vi "Linux parse ip route get.vi"(8 "error in (no error)":errorcluster, 11 "ip route get output":string="192.168.1.5 dev br0 src 192.168.1.100 uid 1000\n     cache") -> (0 "error out":errorcluster, 2 "gw":refnum<class "Generic Network Address.lvclass">, 3 "route ok?":bool)   [LabVIEW 2020, in "NI_WFCN.lvlib" / "IPv4 Network Address.lvclass"]
doc: "Linux: Parse the output of `ip route get $ip` to determine if an address is routable."
uses:
  <vilib>/net/WFCN/Addressing/IPv4 Network Address/IPv4 Network Address.lvclass
  <vilib>/net/WFCN/Addressing/Generic Network Address/Generic Network Address.lvclass
  <vilib>/net/WFCN/Addressing/IPv4 Network Address/IPv4 Network Address.lvclass/IPv4 Network Address.ctl
  <vilib>/net/WFCN/Addressing/Generic Network Address/Generic Network Address.lvclass/Generic Network Address.ctl
  <vilib>/net/WFCN/Addressing/Hostname Network Address/Hostname Network Address.lvclass/Hostname Network Address.ctl
  <vilib>/net/WFCN/Addressing/Hostname Network Address/Create from string.vi
  <vilib>/net/WFCN/Utility/Is IPv4 address.vi
  <vilib>/net/WFCN/Addressing/IPv4 Network Address/Create from U32.vi
  <vilib>/net/WFCN/Addressing/Generic Network Address/Create for unparsable.vi
  <vilib>/net/WFCN/Utility/Is hostname mDNS.vi
  e:/builds/penguin/labview/branches/2020/dev/dist/vi.lib/net/WFCN/Addressing/Generic Network Address/Generic Network Address.lvclass
  <vilib>/net/WFCN/Addressing/Hostname Network Address/Hostname Network Address.lvclass
  <vilib>/net/WFCN/Addressing/mDNS Hostname Network Address/mDNS Hostname Network Address.lvclass
  e:/builds/penguin/labview/branches/2020/dev/dist/vi.lib/net/WFCN/Addressing/Hostname Network Address/Hostname Network Address.lvclass
  <vilib>/Utility/error.llb/Error Cluster From Error Code.vi
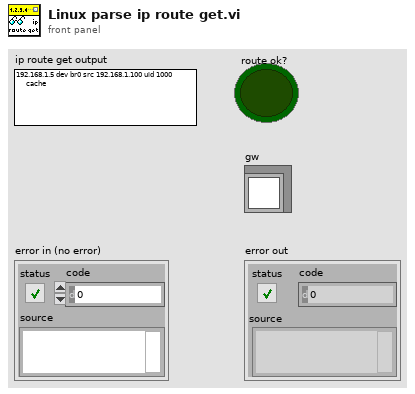
[diagram p1: front panel]
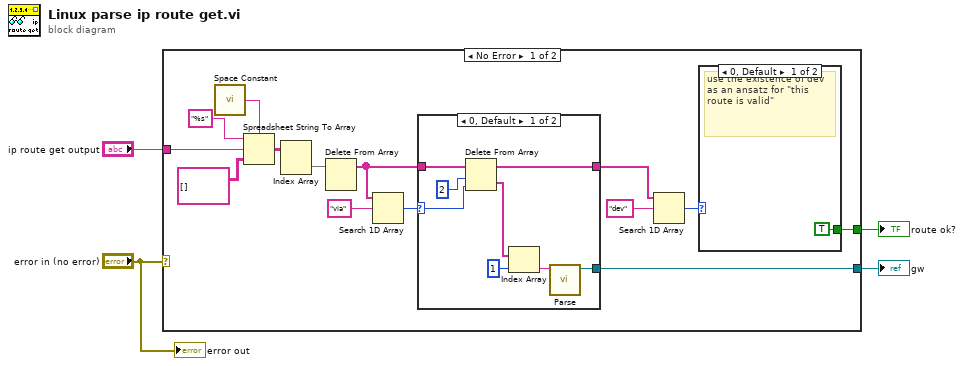
[diagram p0: block diagram]
diagram:
  n1 = case shown="No Error" "error in (no error)" {
    tunnel: "ip route get output" -> [w18 _]
    tunnel: [w6 _] -> w3
    tunnel: [w5 _] -> w2
    frame No Error {
      n2 = call <vilib>:"Space Constant.vi"() -> ("String"=w17:string)
      n3 = Spreadsheet String To Array(delimiter (Tab)=w17, format string="%s", spreadsheet string=w18, array type (2D Dbl)=string[][] []) -> (array=w14:string[][])
      n4 = Index Array(array=w14) -> (element=w12:string[])  [unwired: 2 in]
      n5 = Delete From Array(array=w12) -> (array with subset deleted=w11:string[])  [unwired: 2 in, 1 out]
      n6 = Search 1D Array(1D array=w11, element="via") -> (index of element=w10:i32)  [unwired: 1 in]
      n7 = case shown="0, Default" w10 {
        selector: w10 -> [w26 _]
        tunnel: w11 -> [w27 w28]
        tunnel: [w24 w28] -> w7
        tunnel: [w20 _] -> w6
        frame 0, Default {
          n8 = Delete From Array(array=w27, length=2, index=w26) -> (deleted portion=w22:string[], array with subset deleted=w24:string[])
          n9 = Index Array(array=w22, index=1) -> (element=w21:string)
          n10 = call <vilib>:"Parse.vi"("address string"=w21) -> ("address"=w20:refnum<class "Generic Network Address.lvclass">)  [unwired: 10 in]
        }
        frame -1 {
        }
      }
      n11 = Search 1D Array(1D array=w7, element="dev") -> (index of element=w9:i32)  [unwired: 1 in]
      n12 = case shown="0, Default" w9 {
        tunnel: [TRUE _] -> w5
        frame 0, Default {
          # "use the existence of dev as an ansatz for \"this route is valid\""
        }
        frame -1 {
        }
      }
    }
    frame Error {
    }
  }
  "gw" <- w3
  "route ok?" <- w2
  "error out" <- "error in (no error)"
